vi "反控数据上传(子VI).vi"(8 "error in (no error)":errorcluster caption="错误输入（无错误）", 11 "QN":string) -> (0 "error out":errorcluster caption="错误输出")   [LabVIEW 2016, in "数据传输系统-04.lvlib"]
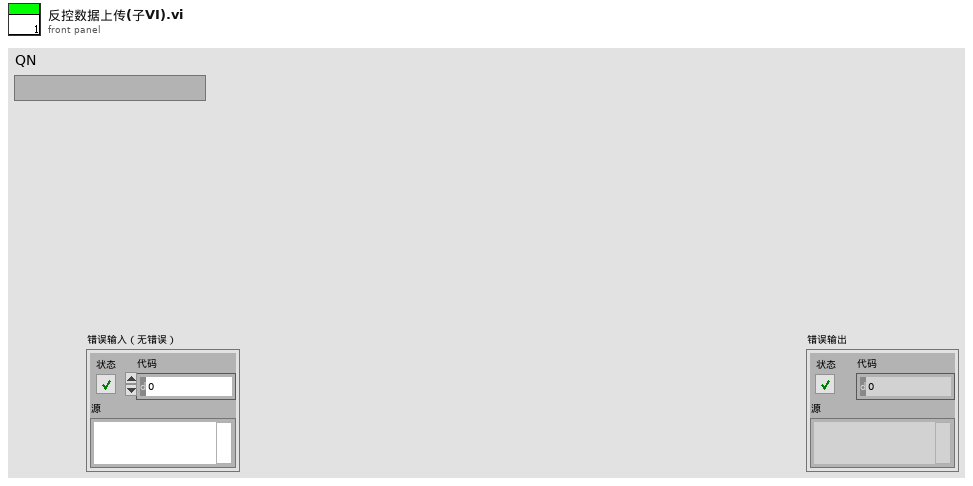
[diagram p1: front panel]
types:
  T1 = cluster{"setini":string, "sysini":string, "hechaini":string, "actualwrite":string, "actualread":string, "datasent":string, "反控命令信息队列":string, "反控与仪器交互":string}
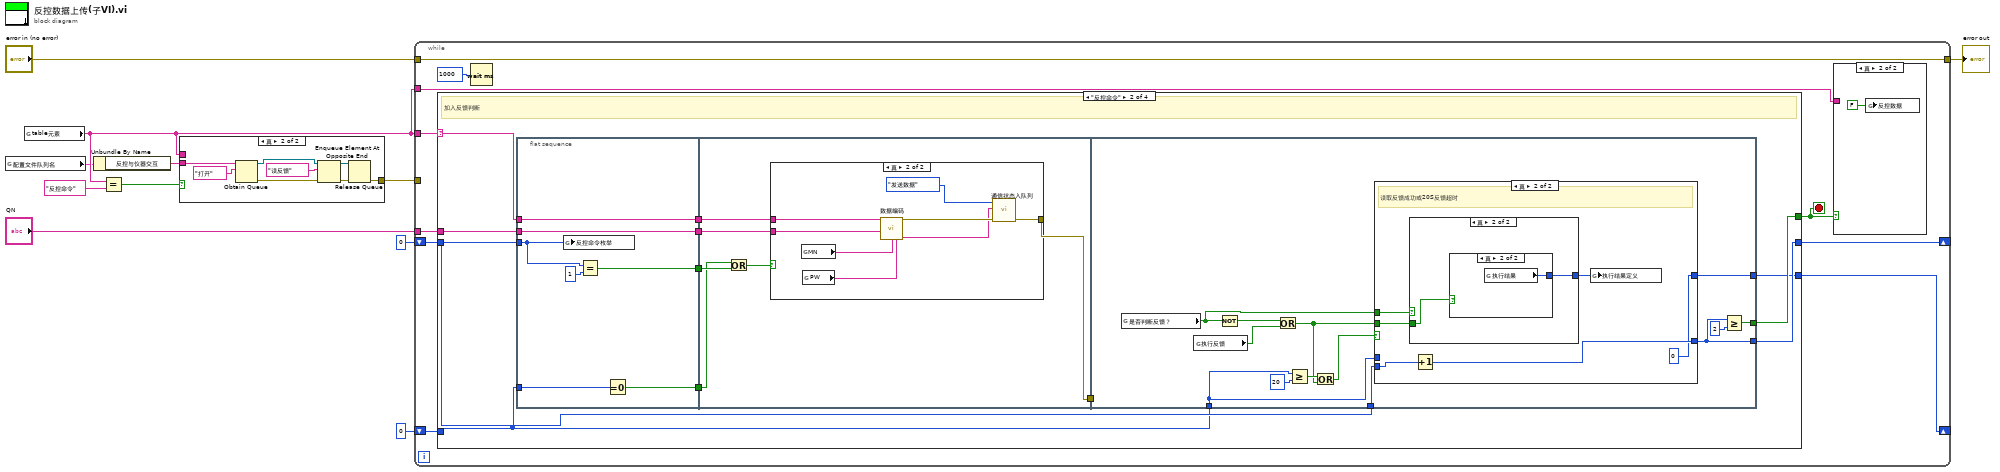
[diagram p0: block diagram]
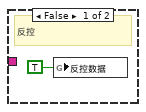
[diagram p3: hidden frame]
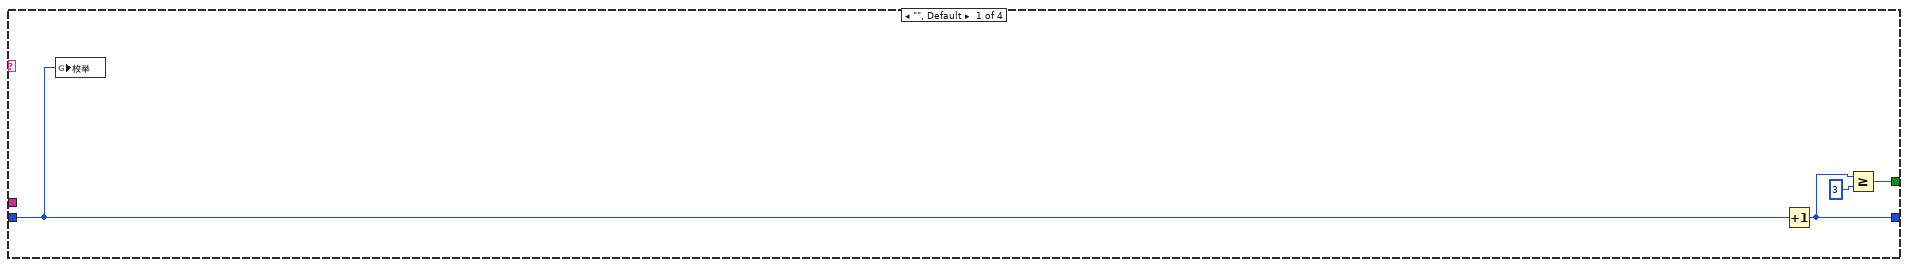
[diagram p4: hidden frame]
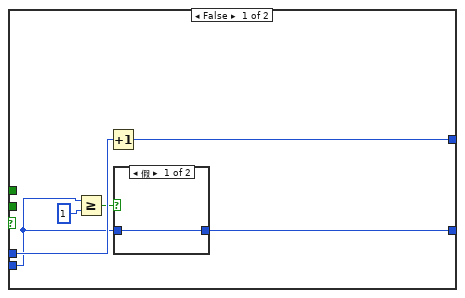
[diagram p6: hidden frame]
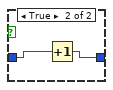
[diagram p7: hidden frame]
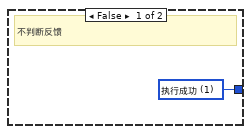
[diagram p8: hidden frame]
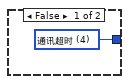
[diagram p9: hidden frame]
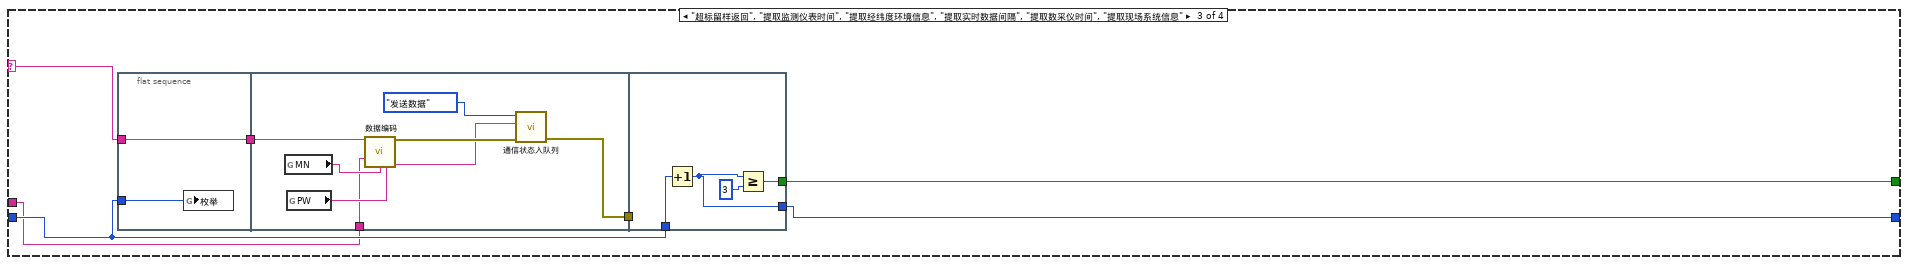
[diagram p10: hidden frame]
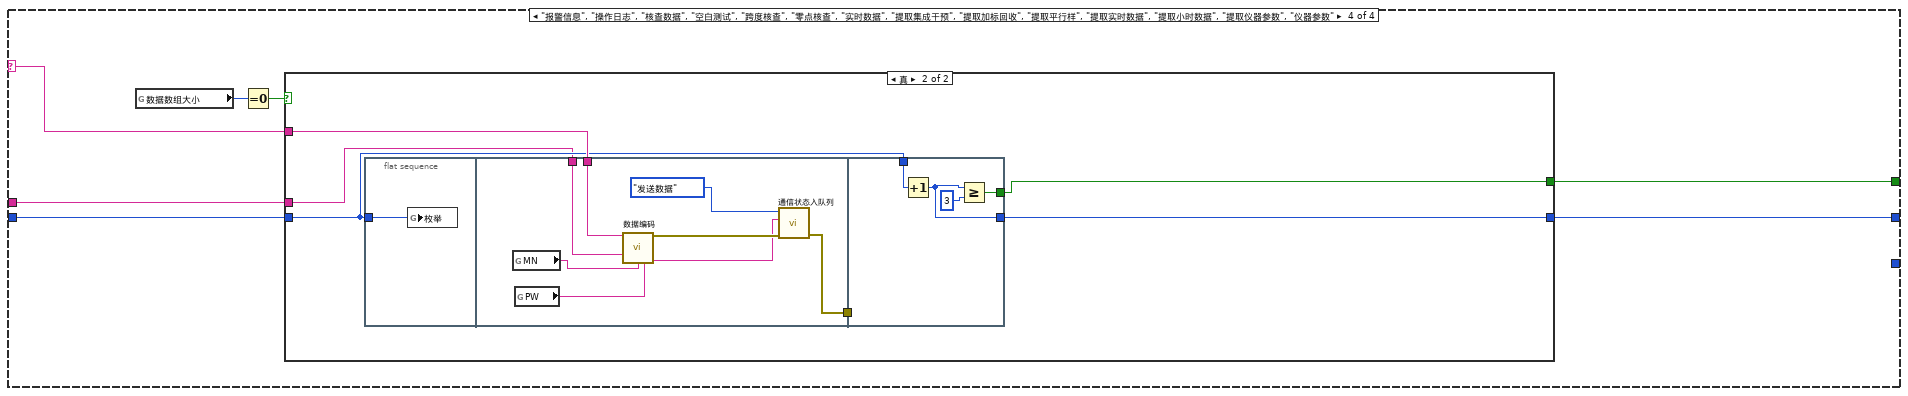
[diagram p11: hidden frame]
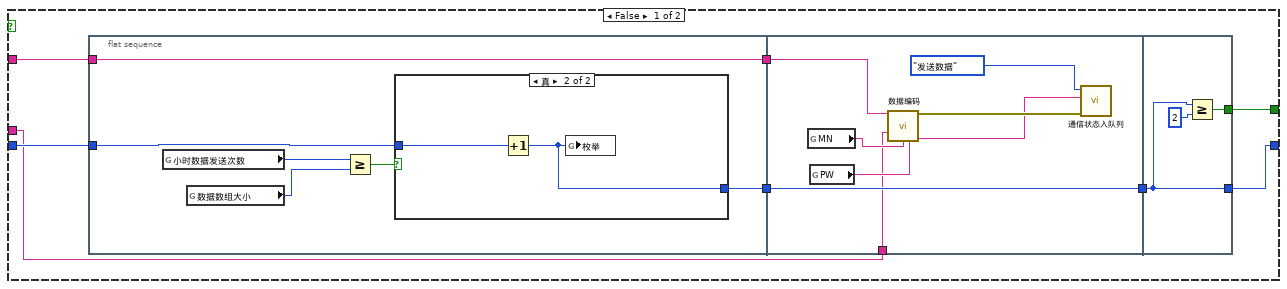
[diagram p12: hidden frame]
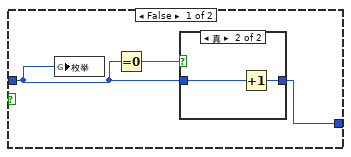
[diagram p13: hidden frame]
diagram:
  n1 = global read "断电保存全局.vi" "配置文件队列名"() -> (w2:T1)
  n2 = global read "全局1.vi" "table元素"() -> (w4:string)
  n3 = Unbundle By Name(w2) -> ("反控与仪器交互"=w1:string)
  n4 = Equal?(x=w4, y="反控命令") -> (x = y?=w3:bool)
  n5 = case shown="真" w3 {
    tunnel: [_ w13] -> w7
    tunnel: w4 -> [_ _]
    tunnel: w1 -> [_ w12]
    frame False {
    }
    frame True {
      n6 = Obtain Queue(name (unnamed)=w12, element data type="打开" ("读取写入选择")) -> (queue out=w18:refnum<queue>, error out=w17:errorcluster)  [unwired: 3 in, 1 out]
      n7 = Enqueue Element At Opposite End(queue=w18, element="读反馈" ("读取写入选择"), error in (no error)=w17) -> (queue out=w15:refnum<queue>, error out=w14:errorcluster)  [unwired: 1 in, 1 out]
      n8 = Release Queue(queue=w15, error in (no error)=w14) -> (error out=w13:errorcluster)  [unwired: 1 in, 2 out]
    }
  }
  n9 = while {
    tunnel: w4 -> [w29]
    shift-right: [w27] -> _
    shift-left: 0 -> [w28]
    tunnel: w4 -> [w25]
    tunnel: "QN" -> [w23]
    tunnel: "error in (no error)" -> [w22]
    tunnel: [w22] -> w8
    tunnel: w7 -> [_]
    shift-right: [w20] -> _
    shift-left: 0 -> [w21]
    stop <- w26 stop-if-true
    n10 = case shown="\"反控命令\"" w29 {
      selector: w29 -> [_ w44 w108 w125]
      tunnel: w28 -> [w34 w45 w105 w124]
      tunnel: [w33 w42 w104 w129] -> w26
      tunnel: [w32 w43 w103 w128] -> w27
      tunnel: w23 -> [_ w41 w102 w123]
      tunnel: w21 -> [_ w37 _ _]
      tunnel: [_ w39 _ _] -> w20
      frame "", Default {
        n11 = global write "全局1.vi" "枚举"(w34) -> ()
        n12 = Increment(x=w34) -> (x+1=w32:i32)
        n13 = Greater Or Equal?(x=w32, y=3) -> (x >= y?=w33:bool)
      }
      frame "反控命令" {
        # "加入反馈判断"
        n14 = flat-sequence {
          tunnel: w44 -> [w54]
          tunnel: [w54] -> w47
          tunnel: w45 -> [w52]
          tunnel: w41 -> [w53]
          tunnel: [w53] -> w40
          tunnel: [w50] -> w38
          tunnel: w37 -> [w49]
          tunnel: [w48] -> w36
          tunnel: w47 -> [w60]
          tunnel: [w59] -> w46
          tunnel: w40 -> [w58]
          tunnel: w38 -> [w56]
          tunnel: w36 -> [w55]
          tunnel: w46 -> [_]
          tunnel: w45 -> [w80]
          tunnel: [w79] -> w42
          tunnel: [w78] -> w43
          tunnel: w37 -> [w76]
          tunnel: [w77] -> w39
          frame #0 {
            n15 = global write "全局 反控命令枚举.vi" "反控命令枚举"(w52) -> ()
            n16 = Equal?(x=w52, y=1) -> (x = y?=w50:bool)
            n17 = Equal To 0?(x=w49) -> (x = 0?=w48:bool)
          }
          frame #1 {
            n18 = Or(x=w55, y=w56) -> (x .or. y?=w57:bool)
            n19 = case shown="真" w57 {
              tunnel: w60 -> [_ w65]
              tunnel: [_ w64] -> w59
              tunnel: w58 -> [_ w63]
              frame False {
              }
              frame True {
                n20 = global read "断电保存全局.vi" "MN"() -> (w68:string)
                n21 = global read "断电保存全局.vi" "PW"() -> (w67:string)
                n22 = call "数据编码.vi"("table输入"=w65, "QN"=w63, "MN"=w68, "PW"=w67) -> ("错误常量"=w66:errorcluster, "通讯包字符串"=w61:string)  [unwired: 10 in]
                n23 = call "通信状态入队列.vi"("错误输入（无错误）"=w66, "发送报文"=w61, "枚举"=enum16{"打开连接", "发送数据", "读取数据", "数据处理", "关闭连接"}."发送数据") -> ("错误输出"=w64:errorcluster)  [unwired: 8 in]
              }
            }
          }
          frame #2 {
            n24 = global read "全局 反控命令枚举.vi" "是否判断反馈？"() -> (w69:bool)
            n25 = global read "全局 反控命令枚举.vi" "执行反馈"() -> (w72:bool)
            n26 = Not(x=w69) -> (.not. x?=w70:bool)
            n27 = Or(x=w70, y=w72) -> (x .or. y?=w71:bool)
            n28 = Greater Or Equal?(x=w76, y=20) -> (x >= y?=w73:bool)
            n29 = Or(x=w73, y=w71) -> (x .or. y?=w74:bool)
            n30 = case shown="真" w74 {
              tunnel: w80 -> [w83 w96]
              tunnel: [w82 w95] -> w78
              tunnel: w76 -> [w87 _]
              tunnel: [w86 0] -> w77
              tunnel: w71 -> [_ w94]
              tunnel: w69 -> [_ w92]
              frame False {
                n31 = Greater Or Equal?(x=w83, y=1) -> (x >= y?=w84:bool)
                n32 = Increment(x=w87) -> (x+1=w86:i32)
                n33 = case shown="假" w84 {
                  tunnel: w83 -> [w88 w90]
                  tunnel: [w88 w89] -> w82
                  frame False {
                  }
                  frame True {
                    n34 = Increment(x=w90) -> (x+1=w89:i32)
                  }
                }
              }
              frame True {
                # "读取反馈成功或20S反馈超时"
                n35 = case shown="真" w92 {
                  tunnel: w94 -> [_ w99]
                  tunnel: [w97 w98] -> w91
                  frame False {
                    w97 = u16 1 items=["执行成功"=1, "执行失败，但不知道原因"=2, "命令请求条件错误"=3, "通讯超时"=4, "系统繁忙不能执行"=5, "系统故障"=6, "没有数据"=100] ("执行结果定义")
                    # "不判断反馈"
                  }
                  frame True {
                    n36 = case shown="真" w99 {
                      tunnel: [w100 w101] -> w98
                      frame False {
                        w100 = u16 4 items=["执行成功"=1, "执行失败，但不知道原因"=2, "命令请求条件错误"=3, "通讯超时"=4, "系统繁忙不能执行"=5, "系统故障"=6, "没有数据"=100] ("执行结果定义")
                      }
                      frame True {
                        n37 = global read "全局 反控命令枚举.vi" "执行结果"() -> (w101:u16)
                      }
                    }
                  }
                }
                n38 = Increment(x=w96) -> (x+1=w95:i32)
                n39 = global write "全局 反控命令枚举.vi" "执行结果定义"(w91) -> ()
              }
            }
            n40 = Greater Or Equal?(x=w78, y=2) -> (x >= y?=w79:bool)
          }
        }
      }
      frame "超标留样返回", "提取监测仪表时间", "提取经纬度环境信息", "提取实时数据间隔", "提取数采仪时间", "提取现场系统信息" {
        n41 = flat-sequence {
          tunnel: w108 -> [w110]
          tunnel: [w110] -> w107
          tunnel: w105 -> [w109]
          tunnel: w107 -> [w115]
          tunnel: [w114] -> w106
          tunnel: w102 -> [w113]
          tunnel: w106 -> [_]
          tunnel: w105 -> [w121]
          tunnel: [w120] -> w104
          tunnel: [w119] -> w103
          frame #0 {
            n42 = global write "全局1.vi" "枚举"(w109) -> ()
          }
          frame #1 {
            n43 = global read "断电保存全局.vi" "MN"() -> (w118:string)
            n44 = global read "断电保存全局.vi" "PW"() -> (w117:string)
            n45 = call "数据编码.vi"("table输入"=w115, "QN"=w113, "MN"=w118, "PW"=w117) -> ("错误常量"=w116:errorcluster, "通讯包字符串"=w111:string)  [unwired: 10 in]
            n46 = call "通信状态入队列.vi"("错误输入（无错误）"=w116, "发送报文"=w111, "枚举"=enum16{"打开连接", "发送数据", "读取数据", "数据处理", "关闭连接"}."发送数据") -> ("错误输出"=w114:errorcluster)  [unwired: 8 in]
          }
          frame #2 {
            n47 = Increment(x=w121) -> (x+1=w119:i32)
            n48 = Greater Or Equal?(x=w119, y=3) -> (x >= y?=w120:bool)
          }
        }
      }
      frame "报警信息", "操作日志", "核查数据", "空白测试", "跨度核查", "零点核查", "实时数据", "提取集成干预", "提取加标回收", "提取平行样", "提取实时数据", "提取小时数据", "提取仪器参数", "仪器参数" {
        n49 = global read "全局 数据数组大小.vi" "数据数组大小"() -> (w127:i32)
        n50 = Equal To 0?(x=w127) -> (x = 0?=w126:bool)
        n51 = case shown="真" w126 {
          tunnel: [w134 w164] -> w129
          tunnel: [w133 w165] -> w128
          tunnel: w125 -> [w132 w167]
          tunnel: w124 -> [w131 w166]
          tunnel: w123 -> [w130 w163]
          frame False {
            n52 = flat-sequence {
              tunnel: w131 -> [w140]
              tunnel: [w138] -> w137
              tunnel: w132 -> [w139]
              tunnel: [w139] -> w136
              tunnel: w137 -> [w159]
              tunnel: [w159] -> w135
              tunnel: w136 -> [w155]
              tunnel: w130 -> [w154]
              tunnel: w135 -> [w162]
              tunnel: [w162] -> w133
              tunnel: [w161] -> w134
              frame #0 {
                n53 = global read "全局 小时数据发送次数.vi" "小时数据发送次数"() -> (w142:i32)
                n54 = global read "全局 数据数组大小.vi" "数据数组大小"() -> (w143:i32)
                n55 = Greater Or Equal?(x=w142, y=w143) -> (x >= y?=w141:bool)
                n56 = case shown="真" w141 {
                  tunnel: w140 -> [w145 w151]
                  tunnel: [w146 w150] -> w138
                  frame False {
                    n57 = global write "全局1.vi" "枚举"(w145) -> ()
                    n58 = Equal To 0?(x=w145) -> (x = 0?=w144:bool)
                    n59 = case shown="真" w144 {
                      tunnel: w145 -> [w147 w149]
                      tunnel: [w147 w148] -> w146
                      frame False {
                      }
                      frame True {
                        n60 = Increment(x=w149) -> (x+1=w148:i32)
                      }
                    }
                  }
                  frame True {
                    n61 = Increment(x=w151) -> (x+1=w150:i32)
                    n62 = global write "全局1.vi" "枚举"(w150) -> ()
                  }
                }
              }
              frame #1 {
                n63 = global read "断电保存全局.vi" "MN"() -> (w156:string)
                n64 = global read "断电保存全局.vi" "PW"() -> (w157:string)
                n65 = call "数据编码.vi"("table输入"=w155, "QN"=w154, "MN"=w156, "PW"=w157) -> ("错误常量"=w158:errorcluster, "通讯包字符串"=w152:string)  [unwired: 10 in]
                n66 = call "通信状态入队列.vi"("错误输入（无错误）"=w158, "发送报文"=w152, "枚举"=enum16{"打开连接", "发送数据", "读取数据", "数据处理", "关闭连接"}."发送数据") -> ()  [unwired: 8 in, 1 out]
              }
              frame #2 {
                n67 = Greater Or Equal?(x=w162, y=2) -> (x >= y?=w161:bool)
              }
            }
          }
          frame True {
            n68 = flat-sequence {
              tunnel: w166 -> [w169]
              tunnel: [w174] -> w168
              tunnel: w167 -> [w173]
              tunnel: w163 -> [w172]
              tunnel: w168 -> [_]
              tunnel: [w180] -> w164
              tunnel: [w179] -> w165
              tunnel: w166 -> [w178]
              frame #0 {
                n69 = global write "全局1.vi" "枚举"(w169) -> ()
              }
              frame #1 {
                n70 = global read "断电保存全局.vi" "MN"() -> (w177:string)
                n71 = global read "断电保存全局.vi" "PW"() -> (w176:string)
                n72 = call "数据编码.vi"("table输入"=w173, "QN"=w172, "MN"=w177, "PW"=w176) -> ("错误常量"=w175:errorcluster, "通讯包字符串"=w170:string)  [unwired: 10 in]
                n73 = call "通信状态入队列.vi"("错误输入（无错误）"=w175, "发送报文"=w170, "枚举"=enum16{"打开连接", "发送数据", "读取数据", "数据处理", "关闭连接"}."发送数据") -> ("错误输出"=w174:errorcluster)  [unwired: 8 in]
              }
              frame #2 {
                n74 = Increment(x=w178) -> (x+1=w179:i32)
                n75 = Greater Or Equal?(x=w179, y=3) -> (x >= y?=w180:bool)
              }
            }
          }
        }
      }
    }
    n76 = Wait (ms)(milliseconds to wait=u32 1000 ("等待时间（毫秒）")) -> ()  [unwired: 1 out]
    n77 = case shown="真" w26 {
      tunnel: w25 -> [_ _]
      frame False {
        # "反控"
        n78 = global write "全局1.vi" "反控数据"(TRUE ("反控数据")) -> ()
      }
      frame True {
        n79 = global write "全局1.vi" "反控数据"(FALSE ("反控数据")) -> ()
      }
    }
  }
  "error out" <- w8
